vi "Just try State machine 16.04.25.vi"() -> ()   [LabVIEW 2020]
panel:
  out "o/p":dbl
  in  "stop":bool
  in  "OK Button":bool
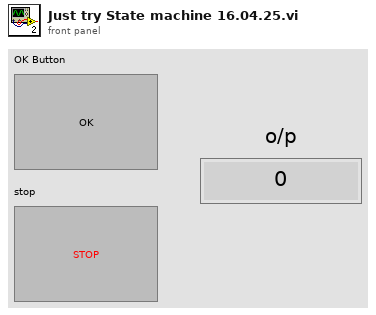
[diagram p1: front panel]
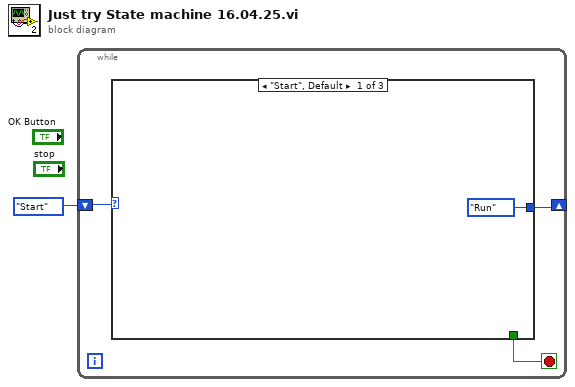
[diagram p0: block diagram]
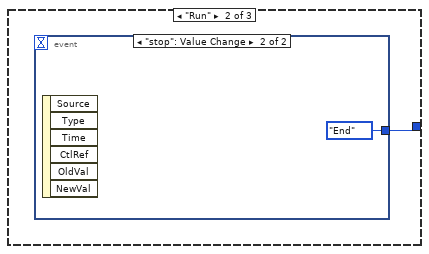
[diagram p2: hidden frame]
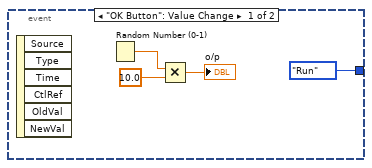
[diagram p3: hidden frame]
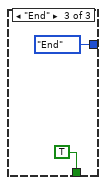
[diagram p4: hidden frame]
diagram:
  n1 = while {
    shift-right: [w3] -> _
    shift-left: enum16{"Start", "Run", "End"}."Start" -> [w4]
    stop <- w2 stop-if-true
    n2 = case shown="\"Start\", Default" w4 {
      tunnel: [enum16{"Start", "Run", "End"}."Run" w6 enum16{"Start", "Run", "End"}."End"] -> w3
      tunnel: [_ _ TRUE] -> w2
      frame "Start", Default {
      }
      frame "Run" {
        n3 = event shown="[1] \"stop\": Value Change" {
          selector: _ -> [_ _]
          dyn-events: _ -> [_ _]
          timeout: _ -> [_ _]
          tunnel: [enum16{"Start", "Run", "End"}."Run" enum16{"Start", "Run", "End"}."End"] -> w6
          event "OK Button": Value Change {
            n4 = event-data() -> ()  [unwired: 1 in, 6 out]
            n5 = Random Number (0-1)() -> (number: 0 to 1=w9:dbl)
            n6 = Multiply(x=w9, y=10.0) -> (x*y=→"o/p":dbl)
          }
          event "stop": Value Change {
            n7 = event-data() -> ()  [unwired: 1 in, 6 out]
          }
        }
      }
      frame "End" {
      }
    }
  }
